vi "NRZ encoder.vi"(8 "Error In":errorcluster, 10 "Bit stream in":u8[](array[numeric])) -> (0 "error out":errorcluster {"code" format="Error %.0f"}, 2 "Bit stream out (NRZ encode)":u8[](array[numeric]))   [LabVIEW 2019]
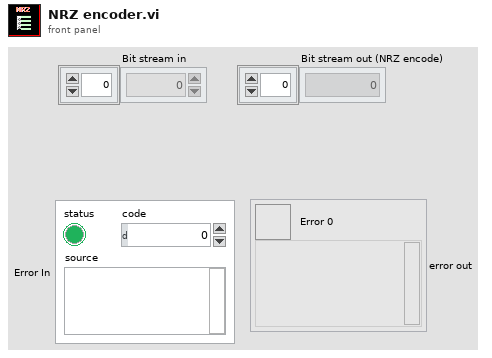
[diagram p1: front panel]
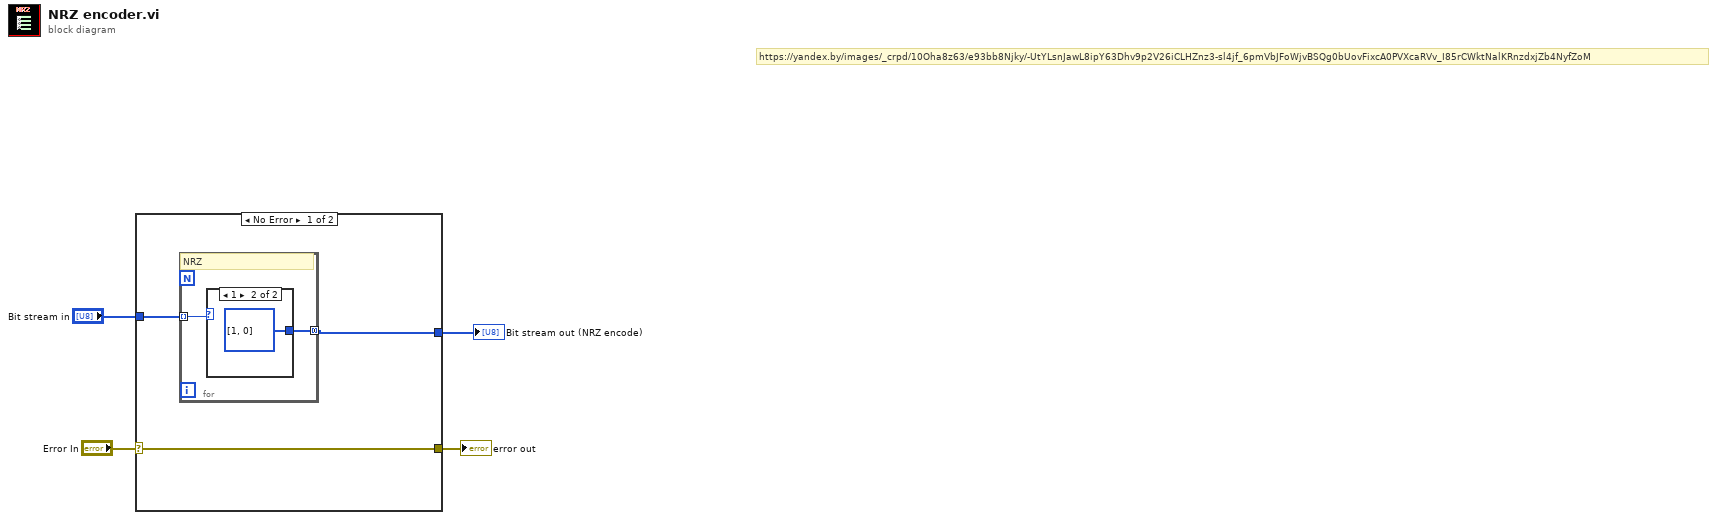
[diagram p0: block diagram]
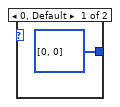
[diagram p2: hidden frame]
diagram:
  # "https://yandex.by/images/_crpd/10Oha8z63/e93bb8Njky/-UtYLsnJawL8ipY63Dhv9p2V26iCLHZnz3-sl4jf_6pmVbJFoWjvBSQg0bUovFixcA0PVXcaRVv_I85rCWktNalKRnzdxjZb4NyfZoM"
  n1 = case shown="No Error" "Error In" {
    selector: "Error In" -> [w7 w12]
    tunnel: "Bit stream in" -> [w6 _]
    tunnel: [w5 _] -> w3
    tunnel: [w7 w12] -> w1
    frame No Error {
      n2 = for {
        tunnel: [w9] -> w5 mode=concatenating
        tunnel: w6 -> [w8] mode=indexing
        # "NRZ"
        n3 = case shown="1" w8 {
          tunnel: [u8[] [0, 0] ("output array") u8[] [1, 0] ("output array")] -> w9
          frame 0, Default {
          }
          frame 1 {
          }
        }
      }
    }
    frame Error {
    }
  }
  "Bit stream out (NRZ encode)" <- w3
  "error out" <- w1
